vi "GlobalDataPointsPerPacket7.vi"() -> ()   [LabVIEW 2013]
panel:
  in  "# Data Points per Packet":i32=9
  # "Each packet is assumed to contain some number\nof data points (given below), each containing 10 bytes,\nplus a two-byte checksum at the end."
  # "For example, if a packet is defined to contain 9 data points,\nit will total 9 x 10 + 2 = 92 total bytes."
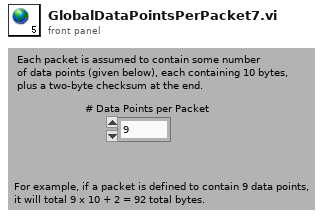
[diagram p1: front panel]
diagram:
